vi "Single Encoder Data.vi"(9 "Tick Constant":dbl, 10 "Rate":dbl, 11 "Distance":dbl) -> (2 "output cluster":T1)   [LabVIEW 2015]
panel:
  in  "single encoder cluster":T1
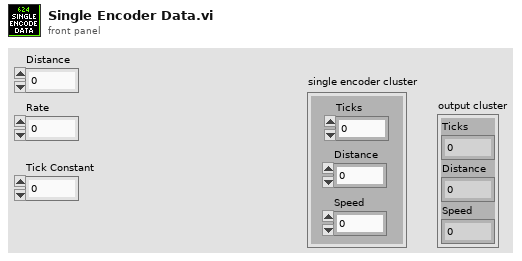
[diagram p1: front panel]
types:
  T1 = cluster{"Ticks":dbl, "Distance":dbl, "Speed":dbl}
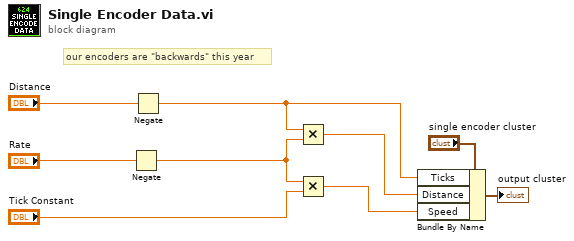
[diagram p0: block diagram]
diagram:
  # "our encoders are \"backwards\" this year"
  n1 = Negate(x="Rate") -> (-x=w1:dbl)
  n2 = Negate(x="Distance") -> (-x=w3:dbl)
  n3 = Multiply(x=w3, y=w1) -> (x*y=w8:dbl)
  n4 = Multiply(x=w1, y="Tick Constant") -> (x*y=w6:dbl)
  n5 = Bundle By Name(cluster="single encoder cluster", "Ticks"=w3, "Distance"=w8, "Speed"=w6) -> (→"output cluster":T1)
